vi "RT Host Globals.vi"() -> ()   [LabVIEW 2020]
doc: "Author: Scott Hannahs <sth@magnet.fsu.edu>\nCopyright 2018 Florida State University, All rights reserved."
panel:
  in  "Mail Relay":string="mailrelay.fsu.edu"
  in  "Trip File Template":string="SCH Trip "
  in  "Log File Template":string="SCH Log "
  in  "System Net Name":string="SCHProtection"
  in  "Notification Email":string="controlroom@magnet.fsu.edu"
  out "Start DateStamp":timestamp format="%<%H:%M:%S%5u\n%Y/%m/%d>T"
  out "Calibration DateStamp":timestamp format="%<%H:%M:%S%5u\n%Y/%m/%d>T"
  out "# Clients":u32
  in  "File Storage command":string="for year in `/bin/ls \"LOGFILE TEMPLATE\"20* | sed -e\"s/LOGFILE TEMPLATE//\" | sed -e\"s/-.*//\" | sort -u` ; do rsync -avz --update --chmod=u=rwX,g=rwX,o=rX --include=\"**/LOGFILE TEMPLATE\"$year\"*.bin\" --exclude=\"*\" . rmps@opsserver.magnet.fsu.edu:\"/Users/Shared/Groups/Operations/Magnet\\ Data/FOLDER\\ Data\\ Files/\"$year\"/Cell\\ 14/\"; done"
  in  "Net Svc Name":string="SCHProtection"
  out "Log File Ref":refnum<file>
  in  "Raw Buffer Size (Secs)":dbl=100.0
  in  "Operator Commands":string[](array[string])=["Reset PS Enable", "Reset Breaker Enable", "Reset", "Cooldown Mode"]
  in  "Comm port":u16=17008
  out "Build":u8
  out "Fix":u8
  out "Minor":u8
  out "Major":u8
  in  "Sec Drop Connection":dbl=120.0
  in  "Total Seconds for Trip File":dbl=40.0
  in  "mS after Trip for File":u32=20000
  in  "Data Size":u32=55
  in  "Raw Data Period":dbl=0.0001024
  in  "Decimation Factor":u32=1024
  # "."
  # "."
  # "."
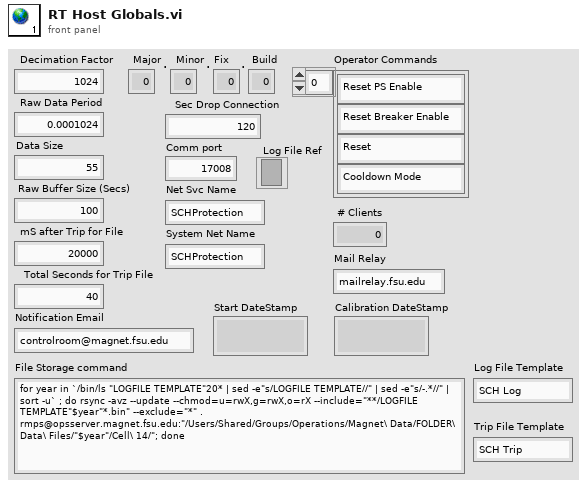
[diagram p1: front panel]
diagram:
